vi "Do.vi"(8 "error in":errorcluster, 10 "Actor in":refnum<class "Actor.lvclass">, 11 "Update Data":refnum<class "Update Controller Data MSG.lvclass">) -> (0 "error out":errorcluster, 2 "Actor out":refnum<class "Actor.lvclass">)   [LabVIEW 2014, in "Controller.lvlib" / "Update Controller Data MSG.lvclass"]
doc: "Writes Data to the Controller Data Map which is contained in a DVR. The message contains two properties - an ID (string) and the data (a Data object). If the ID is not found in the Map, the ID is registered in the IDs portion of the Map."
uses:
  Update Controller Data MSG.lvclass
  <vilib>/ActorFramework/Actor/Actor.lvclass
  Controller.lvclass
  reusable/DAQ Device/Device/Generic Data Update Data MSG/Generic Update Data Message.lvclass/Generic Update Data Message.ctl
  reusable/DAQ Device/Device/Generic Data Update Data MSG/Read Data.vi
  reusable/DAQ Device/Device/Generic Data Update Data MSG/Read ID.vi
  reusable/Data/Data.lvclass
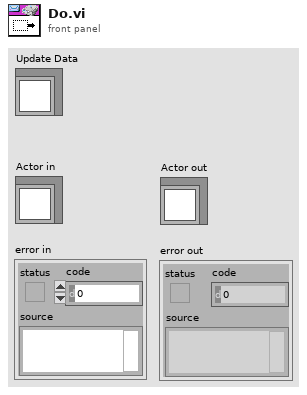
[diagram p1: front panel]
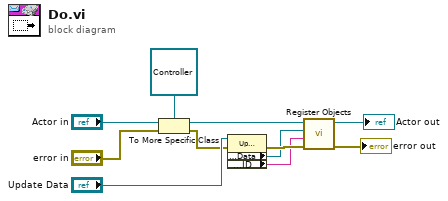
[diagram p0: block diagram]
diagram:
  n1 = To More Specific Class(target class=refnum<class "Controller.lvclass"> refnum ("Controller.lvlib:Controller"), reference="Actor in", error in="error in") -> (specific class reference=w8:refnum<class "Controller.lvclass">, error out=w4:errorcluster)
  n2 = property class="Update Data MSG"(reference="Update Data", error in=w4) -> (error out=w3:errorcluster, "Accessors:Data"=w1:refnum<class "Data.lvclass">, "Accessors:ID"=w2:string)  [unwired: 1 out]
  n3 = call "Register Objects.vi"("error in"=w3, "ID"=w2, "Data"=w1, "Controller in"=w8) -> ("error out"=→"error out":errorcluster, "Controller out"=→"Actor out":refnum<class "Controller.lvclass">)  [unwired: 6 in]
